vi "Serial_AskUserForDeviceCOM.vi"(8 "error in (no error)":errorcluster) -> (0 "error out":errorcluster, 3 "Com-Out":refnum<visa-resource-name>)   [LabVIEW 2020]
panel:
  out "String":string
  in  "Cancel Button":bool
  in  "OK Button":bool
  in  "ComPort Selection":refnum<visa-resource-name>
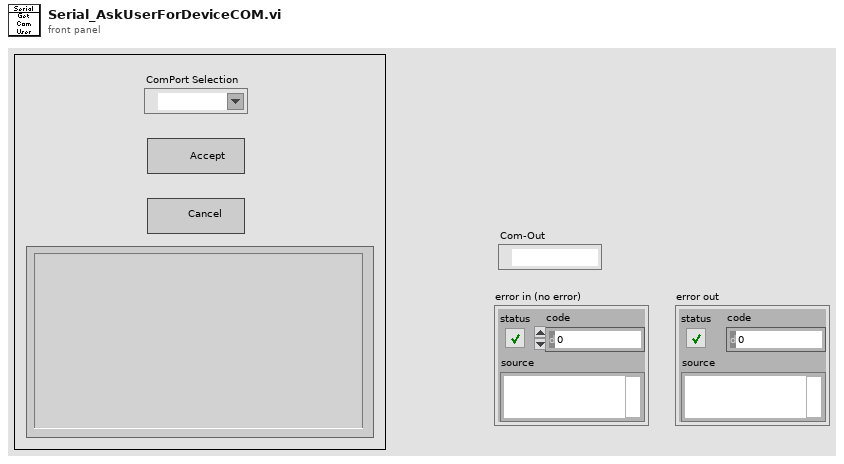
[diagram p1: front panel]
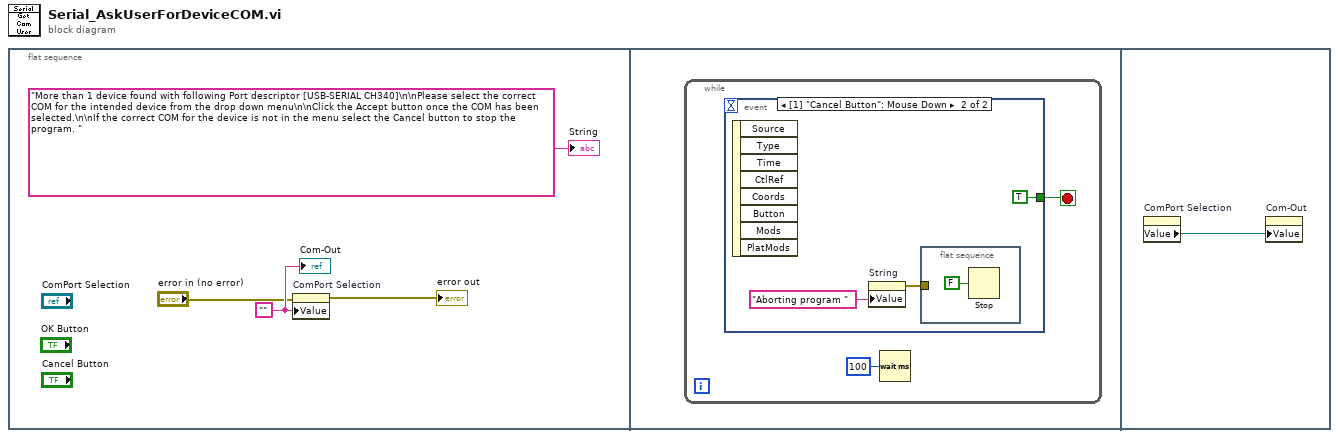
[diagram p0: block diagram]
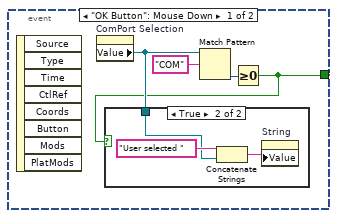
[diagram p2: hidden frame]
diagram:
  n1 = flat-sequence {
    frame #0 {
      w3 = ""
      n2 = property on="ComPort Selection" class="VISAName"(error in="error in (no error)", "Value"=w3) -> (error out=→"error out":errorcluster)  [unwired: 1 in, 1 out]
      "String" <- "More than 1 device found with following Port descriptor [USB-SERIAL CH340]\n\nPlease select the correct COM for the intended device from the drop down menu\n\nClick the Accept button once the COM has been selected.\n\nIf the correct COM for the device is not in the menu select the Cancel button to stop the program. " ("String")
      "Com-Out" <- w3
    }
    frame #1 {
      n3 = while {
        stop <- w5 stop-if-true
        n4 = event shown="[1] \"Cancel Button\": Mouse Down" {
          selector: _ -> [_ _]
          dyn-events: _ -> [_ _]
          timeout: _ -> [_ _]
          tunnel: [w7 TRUE] -> w5
          event "OK Button": Mouse Down {
            n5 = event-data() -> ()  [unwired: 1 in, 8 out]
            n6 = property on="ComPort Selection" class="VISAName"() -> ("Value"=w8:refnum<visa-resource-name>)  [unwired: 2 in, 2 out]
            n7 = Match Pattern(string=w8, regular expression="COM") -> (offset past match=w9:i32)  [unwired: 1 in, 3 out]
            n8 = Greater Or Equal To 0?(x=w9) -> (x >= 0?=w7:bool)
            n9 = case shown="True" w7 {
              tunnel: w8 -> [_ w11]
              frame False {
              }
              frame True {
                n10 = Concatenate Strings("User selected " ("String"), w11) -> (w13:string)
                n11 = property on="String" class="Str"("Value"=w13) -> ()  [unwired: 2 in, 2 out]
              }
            }
          }
          event "Cancel Button": Mouse Down {
            n12 = event-data() -> ()  [unwired: 1 in, 8 out]
            n13 = property on="String" class="Str"("Value"="Aborting program " ("String")) -> (error out=w14:errorcluster)  [unwired: 2 in, 1 out]
            n14 = flat-sequence {
              tunnel: w14 -> [_]
              frame #0 {
                n15 = Stop(stop? (T)=FALSE) -> ()
              }
            }
          }
        }
        n16 = Wait (ms)(milliseconds to wait=u32 100) -> ()  [unwired: 1 out]
      }
    }
    frame #2 {
      n17 = property on="ComPort Selection" class="VISAName"() -> ("Value"=w18:refnum<visa-resource-name>)  [unwired: 2 in, 2 out]
      n18 = property on="Com-Out" class="VISAName"("Value"=w18) -> ()  [unwired: 2 in, 2 out]
    }
  }
